vi "FlatToRichcif_waveformmonitor_Waveform.vi"(5 "OutputClusterType":T1, 11 "InputCluster":T2) -> (3 "OutputCluster":T1)   [LabVIEW 2021, in "CIFWaveformMonitor_server.lvlib"]
uses:
  CIFWaveformMonitor_server.lvlib
  cif_waveformmonitor_Waveform_Flat.ctl
  cif_waveformmonitor_Waveform.ctl
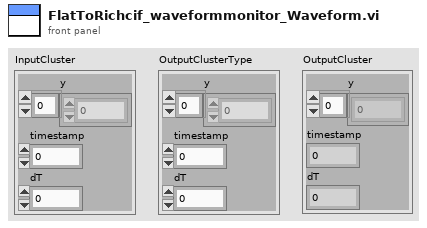
[diagram p1: front panel]
types:
  T1 = typedef "CIFWaveformMonitor_server.lvlib/cif_waveformmonitor_Waveform.ctl" = cluster{"y":dbl[], "timestamp":u64, "dT":dbl}
  T2 = typedef "CIFWaveformMonitor_server.lvlib/cif_waveformmonitor_Waveform_Flat.ctl" = cluster{"y":dbl[], "timestamp":u64, "dT":dbl}
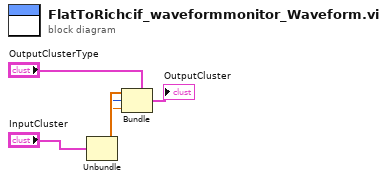
[diagram p0: block diagram]
diagram:
  n1 = Unbundle "Unbundle"("InputCluster") -> ("y"=w3:dbl[], "timestamp"=w2:u64, "dT"=w1:dbl)
  n2 = Bundle "Bundle"(cluster="OutputClusterType", "y"=w3, "timestamp"=w2, "dT"=w1) -> (→"OutputCluster":T1)
